vi "SetParam.vi"(8 "error in (no error)":errorcluster caption="entrée d'erreur (pas d'erreur)", 10 "GaussianRandomProjection":T1={"n_components"="auto", "eps"=0.1, "random_state"=-1} {"random_state" min=-1; "eps" min=0.0}, 11 "GaussianRandomProjection.lvclass":refnum<class "GaussianRandomProjection.lvclass">) -> (0 "error out":errorcluster caption="sortie d'erreur", 3 "GaussianRandomProjection.lvclass":refnum<class "GaussianRandomProjection.lvclass">)   [LabVIEW 2020, in "GaussianRandomProjection.lvclass"]
doc: "Set Parameters"
uses:
  GaussianRandomProjection.lvclass
  GaussianRandomProjection.lvclass/GaussianRandomProjection.ctl
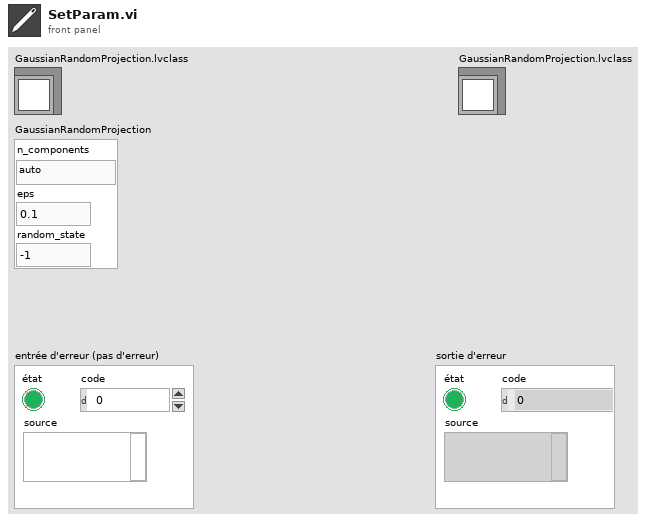
[diagram p1: front panel]
types:
  T1 = cluster{"n_components":string, "eps":dbl, "random_state":i32}
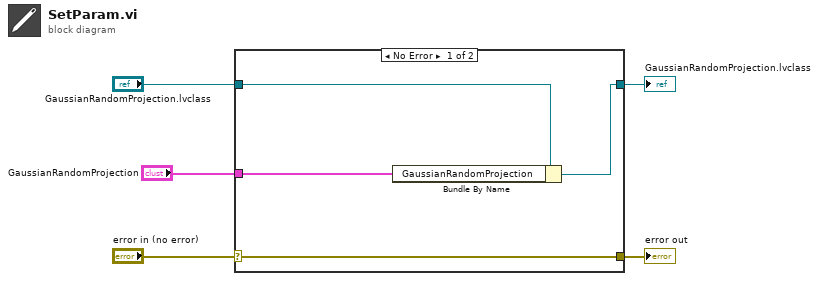
[diagram p0: block diagram]
diagram:
  n1 = case shown="No Error" "error in (no error)" {
    selector: "error in (no error)" -> [w9 w10]
    tunnel: [w9 w10] -> w4
    tunnel: [w7 w11] -> w2
    tunnel: "GaussianRandomProjection.lvclass" -> [w8 w11]
    tunnel: "GaussianRandomProjection" -> [w6 _]
    frame No Error {
      n2 = Bundle By Name(cluster=w8, "GaussianRandomProjection"=w6) -> (w7:refnum<class "GaussianRandomProjection.lvclass">)
    }
    frame Error {
    }
  }
  "error out" <- w4
  "GaussianRandomProjection.lvclass" <- w2
